vi "init.vi"(8 "error in (no error)":errorcluster, 10 "Resource":string, 11 "PsuNiPxi in":refnum<class "PsuNi.lvclass">) -> (0 "error out":errorcluster, 3 "PsuNiPxi out":refnum<class "PsuNi.lvclass">)   [LabVIEW 2023, in "PsuNi.lvclass"]
doc: "<b>Author:</b> Wolfgang\n<b>Description:</b> Method to initialize an instrument by resource name (defined in NI MAX) for any instrument category."
uses:
  PsuNi.lvclass
  <instrlib>/niDCPower/nidcpower.llb/niDCPower Source Mode.ctl
  <instrlib>/niDCPower/nidcpower.llb/niDCPower Output Function.ctl
  PsuNi.lvclass/PsuNi.ctl
  PowerSupply.lvclass
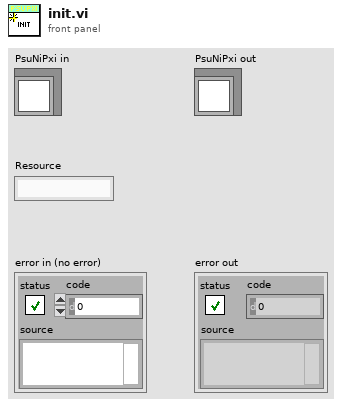
[diagram p1: front panel]
types:
  T1 = typedef "niDCPower Output Function.ctl" = i32
  T2 = typedef "niDCPower Source Mode.ctl" = i32
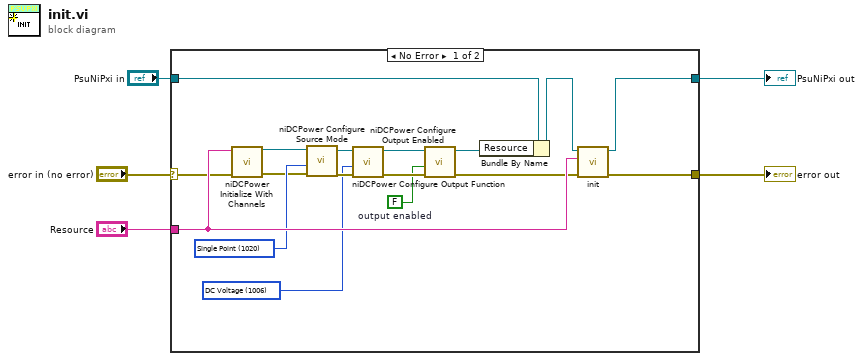
[diagram p0: block diagram]
diagram:
  n1 = case shown="No Error" "error in (no error)" {
    selector: "error in (no error)" -> [w17 w23]
    tunnel: [w22 w23] -> w5
    tunnel: [w21 w24] -> w4
    tunnel: "PsuNiPxi in" -> [w20 w24]
    tunnel: "Resource" -> [w18 _]
    frame No Error {
      w6 = FALSE  # output enabled
      w11 = T1 1006 items=["DC Voltage"=1006, "DC Current"=1007, "Pulse Voltage"=1049, "Pulse Current"=1050] ("output function")
      w15 = T2 1020 items=["Single Point"=1020, "Sequence"=1021] ("source mode")
      n2 = call <instrlib>:"niDCPower Initialize With Channels.vi"("error in (no error)"=w17, "resource name"=w18) -> ("error out"=w12:errorcluster, "instrument handle out"=w16:refnum<k15>)  [unwired: 8 in]
      n3 = call <instrlib>:"niDCPower Configure Source Mode.vi"("error in (no error)"=w12, "source mode"=w15, "instrument handle"=w16) -> ("error out"=w13:errorcluster, "instrument handle out"=w14:refnum<k15>)  [unwired: 7 in]
      n4 = call <instrlib>:"niDCPower Configure Output Function.vi"("error in (no error)"=w13, "output function"=w11, "instrument handle"=w14) -> ("error out"=w8:errorcluster, "instrument handle out"=w9:refnum<k15>)  [unwired: 7 in]
      n5 = call <instrlib>:"niDCPower Configure Output Enabled.vi"("error in (no error)"=w8, "output enabled"=w6, "instrument handle"=w9) -> ("error out"=w7:errorcluster, "instrument handle out"=w10:refnum<k15>)  [unwired: 7 in]
      n6 = Bundle By Name(cluster=w20, "Resource"=w10) -> (w19:refnum<class "PsuNi.lvclass">)
      n7 = call-parent "init.vi"("error in (no error)"=w7, "Resource"=w18, "Instrument in"=w19) -> ("error out"=w22:errorcluster, "Instrument out"=w21:refnum<class "PsuNi.lvclass">)  [unwired: 7 in]
    }
    frame Error {
    }
  }
  "error out" <- w5
  "PsuNiPxi out" <- w4
